vi "gpanel_destroy_ui_events.vi"(8 "error in (no error)":errorcluster, 11 "galvo_panel in":refnum<class "galvo_panel.lvclass">) -> (0 "error out":errorcluster, 3 "galvo_panel out":refnum<class "galvo_panel.lvclass">)   [LabVIEW 2015, in "galvo_panel.lvclass"]
uses:
  galvo_panel.lvclass
  galvo_panel.lvclass/galvo_panel.ctl
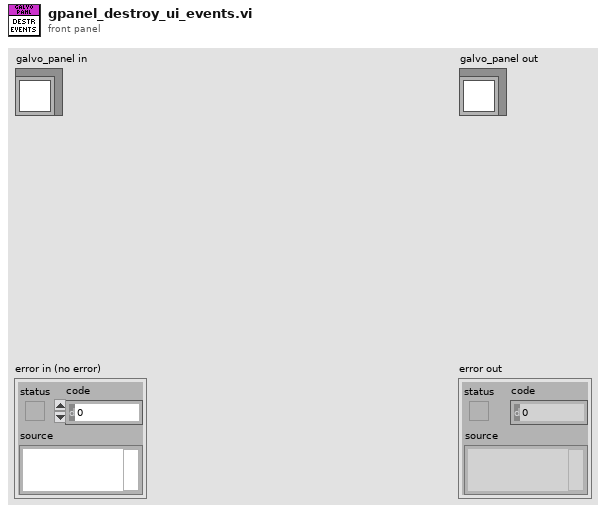
[diagram p1: front panel]
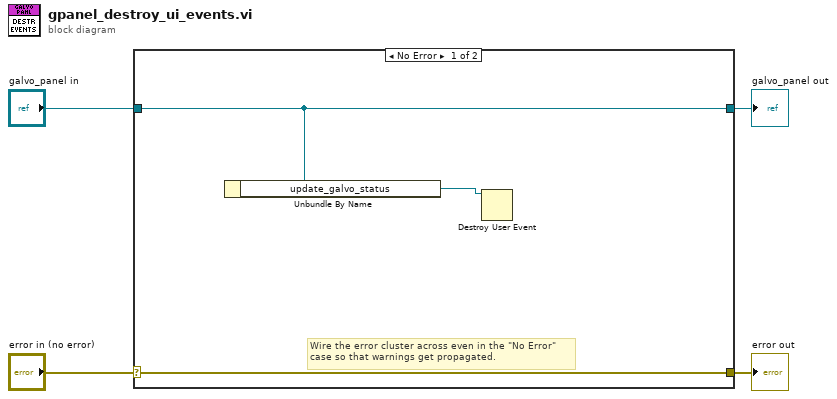
[diagram p0: block diagram]
diagram:
  n1 = case shown="No Error" "error in (no error)" {
    selector: "error in (no error)" -> [w7 w9]
    tunnel: [w7 w9] -> w3
    tunnel: [w6 w8] -> w1
    tunnel: "galvo_panel in" -> [w6 w8]
    frame No Error {
      # "Wire the error cluster across even in the \"No Error\"\ncase so that warnings get propagated."
      n2 = Unbundle By Name(w6) -> ("update_galvo_status"=w5:refnum<user-event>)
      n3 = Destroy User Event(user event=w5) -> ()  [unwired: 1 in, 1 out]
    }
    frame Error {
    }
  }
  "error out" <- w3
  "galvo_panel out" <- w1
